vi "cmc_acquisition.vi"() -> ()   [LabVIEW 2010]
doc: "I. Description:\nThis example demonstrates how to continuously acquire data (waveform) using software timing (rate is governed by while loop iteration interval).\n\nII. Instructions for Running:\n1. Select the physical channel to correspond to where your signal is input on the DAQ device.\n2. Enter the minimum and maximum voltage ranges.\nNote: For better accuracy try to match the input range to the expected voltage level of the measured signal.\n\nIII. Block Diagram Steps:\n1. Create an analog input voltage channel.\n2. Call the Start VI to start the task.\n3. Read the waveform data in a loop until the user hits the stop\nbutton or an error occurs.\n4. Call the Clear Task VI to clear the Task.\n5. Use the popup dialog box to display an error if any.\n\nIV. I/O Connections Overview:\nMake sure your signal input terminal matches the Physical Channel I/O control."
uses:
  <vilib>/Utility/error.llb/DialogType.ctl
  <vilib>/DAQmx/read.llb/DAQmx Read (Analog DBL 1Chan 1Samp).vi
  <vilib>/DAQmx/create/channels.llb/DAQmx Create Channel (AI-Voltage-Basic).vi
  <vilib>/daqmx/miscellaneous.llb/DAQmx Fill In Error Info.vi
panel:
  in  "Load Limit":dbl
  in  "custom scale name":tag
  in  "Write to File":bool
  in  "Software Loop Time (ms)":u32=250
  in  "Physical Channel":tag="Dev1/ai0"
  in  "Minimum Value":dbl=-10.0 format="%0.2f"
  in  "Maximum Value":dbl=10.0 format="%0.2f"
  in  "stop":bool
  out "Measurement":dbl(graph)
  # "For instructions, select Help>>Show Context Help"
  # "Timing Parameters"
  # "Channel Parameters"
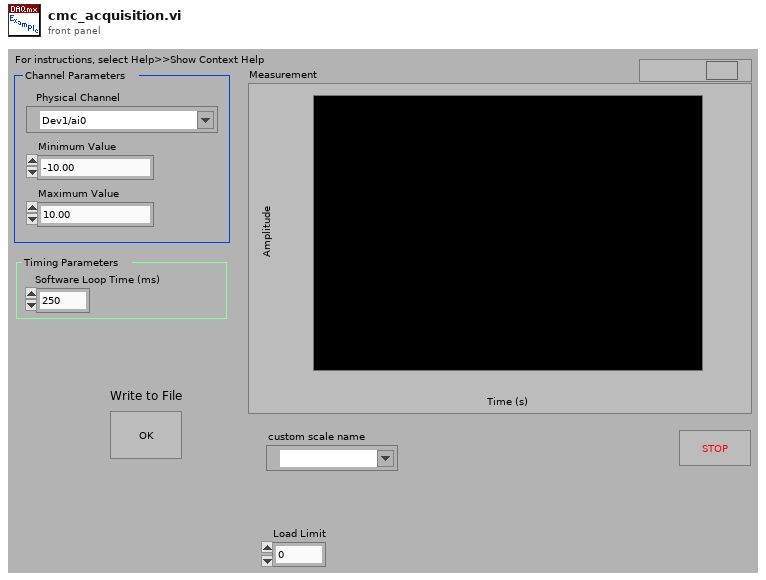
[diagram p1: front panel]
types:
  T1 = enum16{"open", "replace", "create", "open or create", "replace or create", "replace or create with confirmation"}
  T2 = typedef "DialogType.ctl" = u16
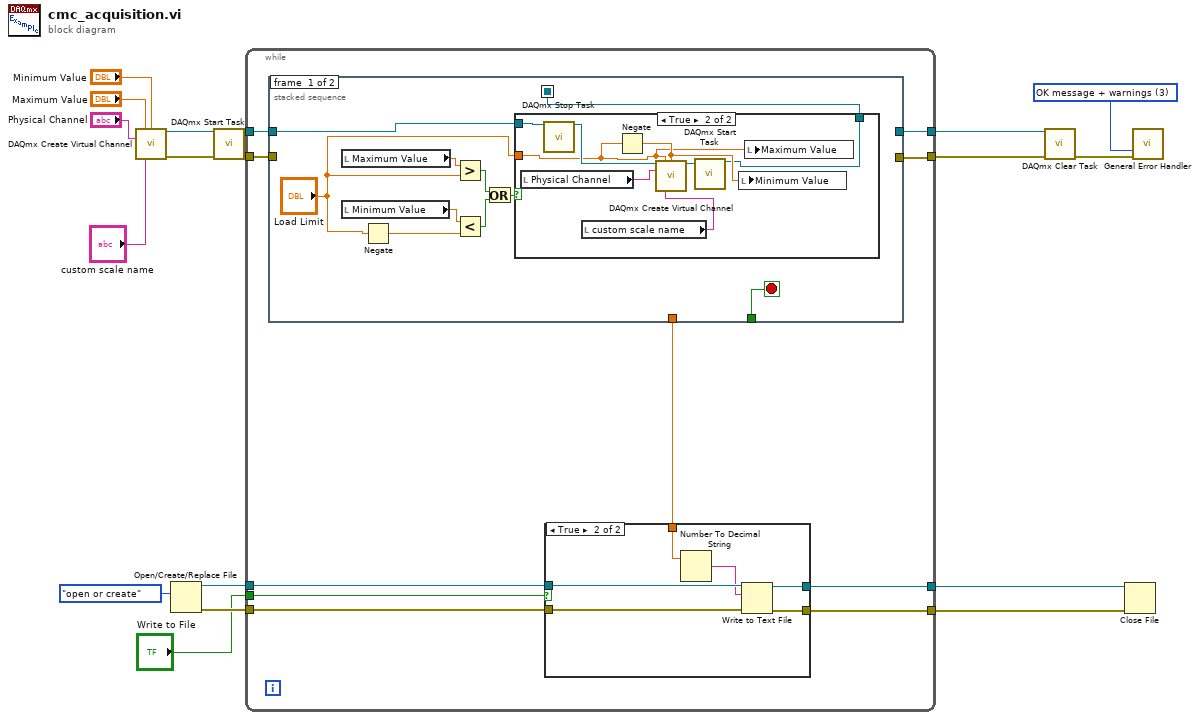
[diagram p0: block diagram]
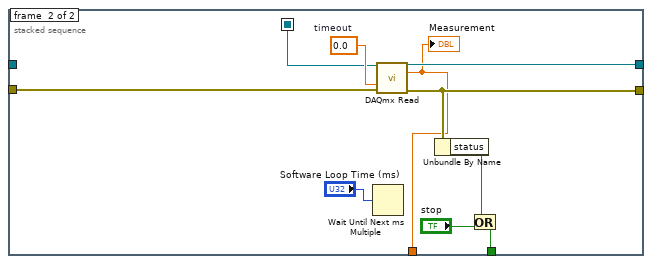
[diagram p3: hidden frame]
diagram:
  w8 = T2 3 items=["no dialog", "OK message", "continue or stop message", "OK message + warnings", "continue/stop + warnings"] ("type of dialog (OK msg:1)")
  n1 = call-poly <vilib>:"DAQmx Create Virtual Channel.vi"("maximum value"="Maximum Value", "minimum value"="Minimum Value", "physical channels"="Physical Channel", "custom scale name"="custom scale name") -> ("task out"=w10:refnum<k21>, "error out"=w9:errorcluster)  [unwired: 10 in]
  n2 = Open/Create/Replace File(operation (0:open)=T1."open or create") -> (refnum out=w6:refnum<file>, error out=w5:errorcluster)  [unwired: 5 in, 1 out]
  n3 = call <vilib>:"DAQmx Start Task.vi"("task/channels in"=w10, "error in"=w9) -> ("task out"=w13:refnum<k21>, "error out"=w16:errorcluster)  [unwired: 12 in]
  n4 = while {
    tunnel: w16 -> [w29]
    tunnel: [w27] -> w15
    tunnel: w13 -> [w19]
    tunnel: [w26] -> w12
    tunnel: w6 -> [w25]
    tunnel: w5 -> [w24]
    tunnel: [w23] -> w4
    tunnel: [w22] -> w3
    tunnel: "Write to File" -> [w21]
    stop <- w28 stop-if-true
    n5 = stacked-sequence {
      seq-local: [w37 _] -> [_ w48]
      tunnel: w29 -> [_ w57]
      tunnel: [_ w56] -> w28
      tunnel: [_ w53] -> w27
      tunnel: [_ w52] -> w26
      tunnel: [_ w49] -> w20
      tunnel: w19 -> [w38 _]
      frame #0 {
        n6 = local read "Maximum Value"() -> (w33:dbl)
        n7 = local read "Minimum Value"() -> (w32:dbl)
        n8 = Negate(x="Load Limit") -> (-x=w30:dbl)
        n9 = Greater?(x=w33, y="Load Limit") -> (0:w35:bool)
        n10 = Less?(x=w32, y=w30) -> (x < y?=w36:bool)
        n11 = Or(x=w35, y=w36) -> (x .or. y?=w34:bool)
        n12 = case shown="True" w34 {
          tunnel: w38 -> [w39 w42]
          tunnel: [w39 w41] -> w37
          tunnel: "Load Limit" -> [_ w40]
          frame False {
          }
          frame True {
            n13 = local read "Physical Channel"() -> (w47:tag)
            n14 = call <vilib>:"DAQmx Stop Task.vi"("task/channels in"=w42) -> ("task out"=w45:refnum<k21>)  [unwired: 13 in, 1 out]
            n15 = local read "custom scale name"() -> (w43:tag)
            n16 = Negate(x=w40) -> (-x=w46:dbl)
            n17 = call-poly <vilib>:"DAQmx Create Virtual Channel.vi"("task in"=w45, "maximum value"=w40, "minimum value"=w46, "physical channels"=w47, "custom scale name"=w43) -> ("task out"=w44:refnum<k21>)  [unwired: 9 in, 1 out]
            n18 = call <vilib>:"DAQmx Start Task.vi"("task/channels in"=w44) -> ("task out"=w41:refnum<k21>)  [unwired: 13 in, 1 out]
            n19 = local write "Minimum Value"(w46) -> ()
            n20 = local write "Maximum Value"(w40) -> ()
          }
        }
      }
      frame #1 {
        w51 = 0.0  # timeout
        n21 = Wait Until Next ms Multiple(millisecond multiple="Software Loop Time (ms)") -> ()  [unwired: 1 out]
        n22 = call-poly <vilib>:"DAQmx Read.vi"("task/channels in"=w48, "timeout"=w51, "error in"=w57) -> ("task out"=w52:refnum<k21>, "data"=w49:dbl, "error out"=w53:errorcluster)  [unwired: 10 in]
        "Measurement" <- w49
        n23 = Unbundle By Name(w53) -> ("status"=w54:bool)
        n24 = Or(x=w54, y="stop") -> (x .or. y?=w56:bool)
      }
    }
    n25 = case shown="True" w21 {
      tunnel: w25 -> [w59 w65]
      tunnel: w24 -> [w58 w64]
      tunnel: [w59 w63] -> w23
      tunnel: [w58 w62] -> w22
      tunnel: w20 -> [_ w61]
      frame False {
      }
      frame True {
        n26 = Number To Decimal String(number=w61) -> (decimal integer string=w60:string)  [unwired: 1 in]
        n27 = Write to Text File(file (use dialog)=w65, text=w60, error in=w64) -> (refnum out=w63:refnum<file>, error out=w62:errorcluster)  [unwired: 1 in, 1 out]
      }
    }
  }
  n28 = call <vilib>:"DAQmx Clear Task.vi"("task in"=w12, "error in"=w15) -> ("error out"=w14:errorcluster)  [unwired: 13 in]
  n29 = Close File(refnum=w4, error in=w3) -> ()  [unwired: 2 out]
  n30 = call <vilib>:"General Error Handler.vi"("type of dialog (OK msg:1)"=w8, "error in (no error)"=w14) -> ()  [unwired: 9 in, 5 out]
